vi "Test 3 Skipped Method.vi"(8 "error in (no error)":errorcluster, 11 "Test Test Case in":refnum<class "Skip Last Test Case.lvclass">) -> (0 "error out":errorcluster, 3 "Test Test Case out":refnum<class "Skip Last Test Case.lvclass">)   [LabVIEW 2020, in "Skip Last Test Case.lvclass"]
uses:
  Skip Last Test Case.lvclass
  source/Framework/Test Case/LUnit Test Case.lvclass
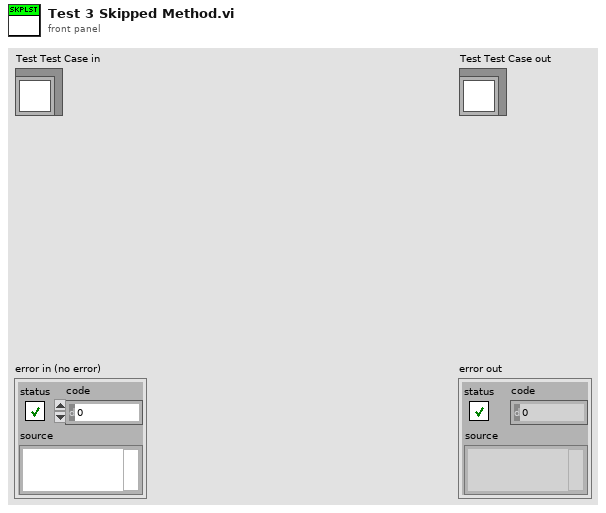
[diagram p1: front panel]
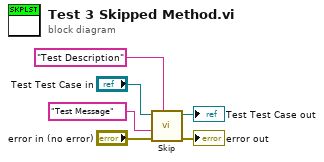
[diagram p0: block diagram]
diagram:
  n1 = call "Skip.vi"("Description"="Test Description", "error in (no error)"="error in (no error)", "Message"="Test Message", "LUnit Test Case In"="Test Test Case in") -> ("error out"=→"error out":errorcluster, "LUnit Test Case Out"=→"Test Test Case out":refnum<class "Skip Last Test Case.lvclass">)  [unwired: 6 in]
